vi "Modify Dequeue Cmds to Requested Node Size.vi"(7 "VI to Code Relative Path":string="IONode\\DLULayer\\Dequeue Cmds From Nodes.vi", 8 "Error In":errorcluster, 10 "NumCasesToAdd":i32=1, 11 "Source Root Path":path=path "C:/Users/kvemishe/Downloads/IONode/DLULayer/Dequeue Cmds From Nodes.vi") -> (0 "Error Out":errorcluster, 1 "Found Object?":bool, 3 "Source Root Path Out":path=path "C:/Users/kvemishe/Downloads/IONode/DLULayer/Dequeue Cmds From Nodes.vi")   [LabVIEW 2014]
doc: "This VI scripts the deque commands VI for the IO Node Engine"
uses:
  <vilib>/Utility/traverseref.llb/TRef TravTarget.ctl
  <vilib>/Utility/traverseref.llb/VI Scripting - Traverse.lvlib
panel:
  out "NumCasesFound":i32
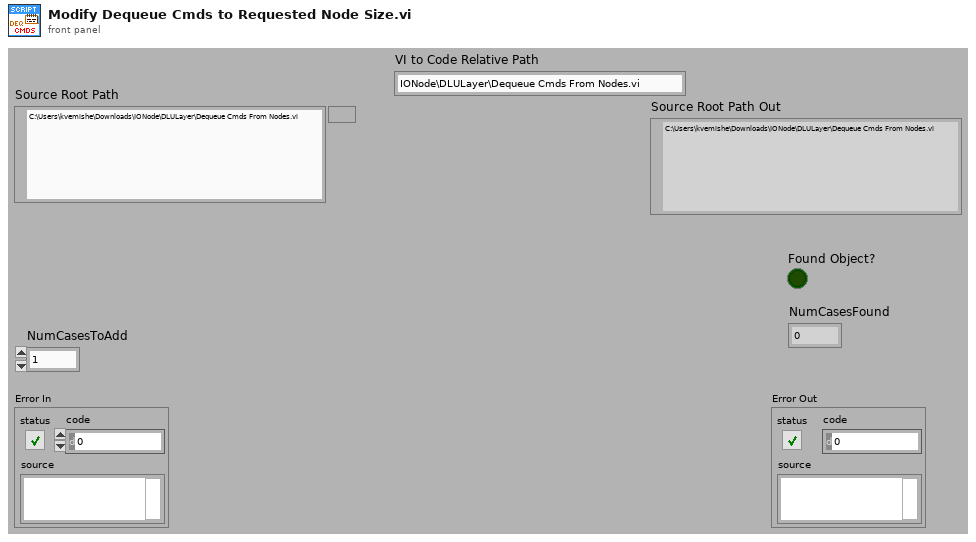
[diagram p1: front panel]
types:
  T1 = typedef "TRef TravTarget.ctl" = enum16{"FP", "BD", "Other"}
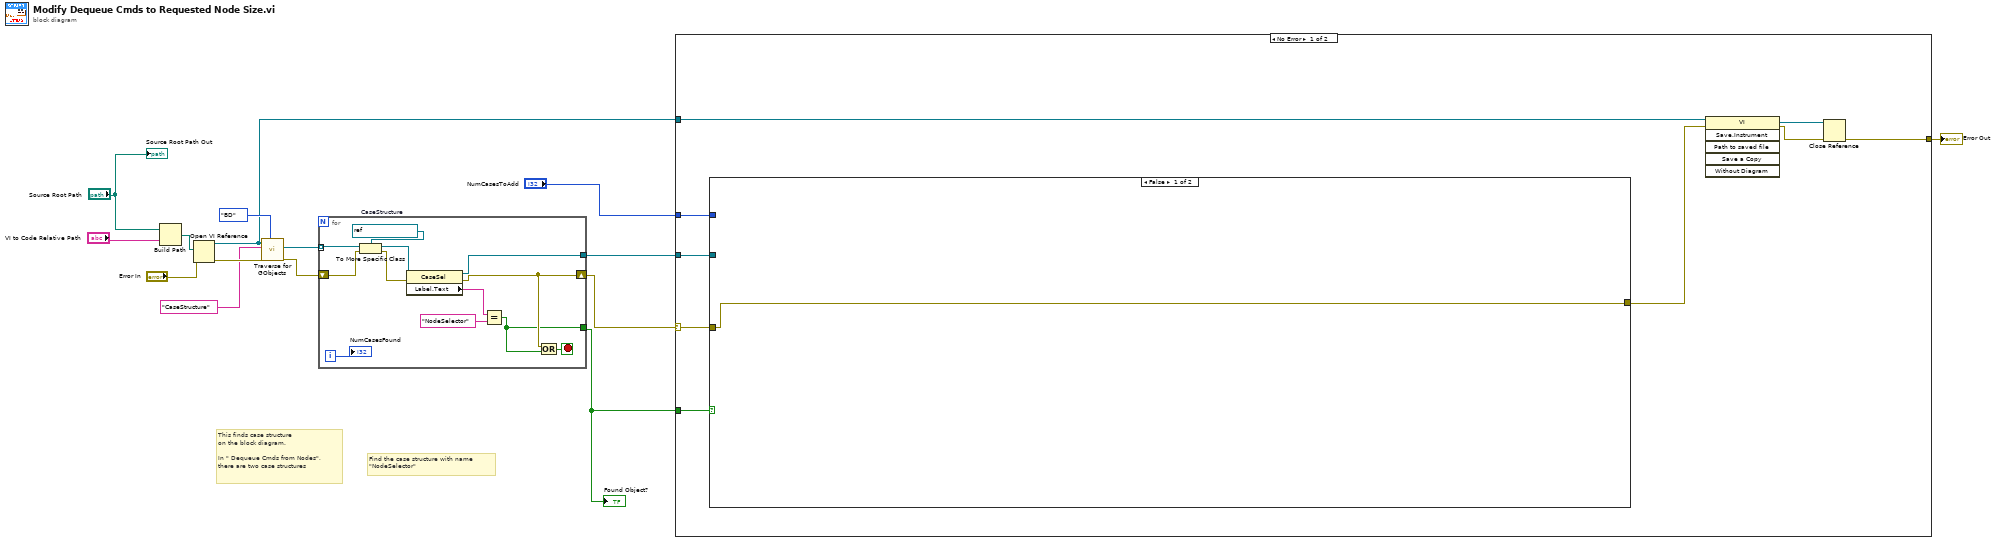
[diagram p0: block diagram]
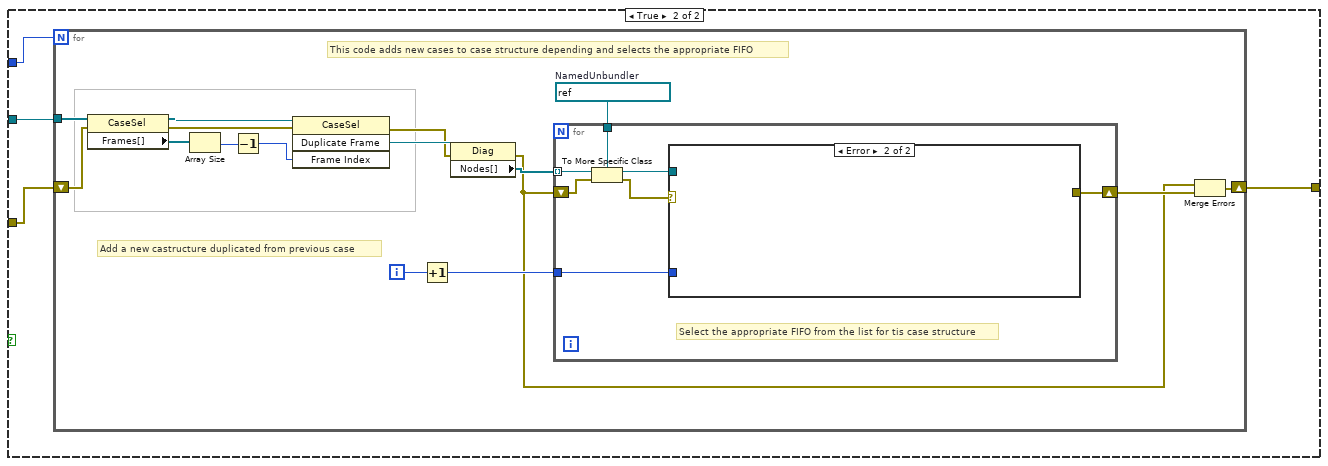
[diagram p2: hidden frame]
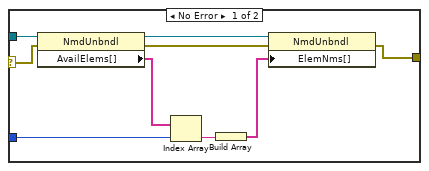
[diagram p3: hidden frame]
diagram:
  # "Find the case structure with name\n\"NodeSelector\""
  # "This finds case structure\non the block diagram.\n\nIn \" Dequeue Cmds from Nodes\",\nthere are two case structures"
  n1 = Build Path(base path="Source Root Path", name or relative path="VI to Code Relative Path") -> (appended path=w3:path)
  n2 = Open VI Reference(vi path=w3, error in (no error)="Error In") -> (vi reference=w6:refnum<vi>, error out=w14:errorcluster)  [unwired: 4 in]
  n3 = call <vilib>:"Traverse for GObjects.vi"("Traverse Target"=TRef_TravTarget."BD", "error in (no error)"=w14, "Class Name"="CaseStructure", "VI Refnum"=w6) -> ("error out"=w11:errorcluster, "References"=w12:refnum<vi>[])  [unwired: 4 in, 2 out]
  n4 = for {
    tunnel: w12 -> [w27] mode=indexing
    shift-right: [w19] -> w9
    shift-left: w11 -> [w25]
    tunnel: [w18] -> w8
    tunnel: [w17] -> w10
    i -> [w16]
    stop <- w20 stop-if-true
    w26 = refnum<vi> refnum  # CaseStructure
    n5 = To More Specific Class(target class=w26, reference=w27, error in=w25) -> (specific class reference=w24:refnum<vi>, error out=w23:errorcluster)
    n6 = property class="CaseSel"(reference=w24, error in=w23) -> (reference out=w17:refnum<vi>, error out=w19:errorcluster, "Label.Text"=w22:string)
    n7 = Equal?(x=w22, y="NodeSelector") -> (x = y?=w18:bool)
    n8 = Or(x=w19, y=w18) -> (x .or. y?=w20:bool)
    "NumCasesFound" <- w16
  }
  "Found Object?" <- w8
  n9 = case shown="No Error" w9 {
    selector: w9 -> [w33 w74]
    tunnel: w10 -> [w36 _]
    tunnel: w8 -> [w35 _]
    tunnel: "NumCasesToAdd" -> [w34 _]
    tunnel: w6 -> [w29 _]
    tunnel: [w28 w74] -> w4
    frame No Error {
      n10 = case shown="False" w35 {
        tunnel: w36 -> [_ w41]
        tunnel: w34 -> [_ w40]
        tunnel: w33 -> [w37 w39]
        tunnel: [w37 w38] -> w30
        frame False {
        }
        frame True {
          n11 = for {
            N: w40 -> [_]
            tunnel: w41 -> [w48]
            shift-right: [w44] -> w38
            shift-left: w39 -> [w45]
            i -> [w47]
            w50 = refnum<vi> refnum  # NamedUnbundler
            # "Add a new castructure duplicated from previous case"
            # "This code adds new cases to case structure depending and selects the appropriate FIFO"
            n12 = property class="CaseSel"(reference=w48, error in=w45) -> (reference out=w57:refnum<vi>, error out=w56:errorcluster, "Frames[]"=w55:refnum<vi>[])
            n13 = Array Size(array=w55) -> (size(s)=w54:i32)
            n14 = Decrement(x=w54) -> (x-1=w53:i32)
            n15 = invoke class="CaseSel" method="Duplicate Frame"(reference=w57, error in=w56, "Frame Index"=w53) -> (error out=w46:errorcluster, "Duplicate Frame"=w52:refnum<vi>)  [unwired: 1 in, 2 out]
            n16 = Increment(x=w47) -> (x+1=w49:i32)
            n17 = property class="Diag"(reference=w52, error in=w46) -> (error out=w42:errorcluster, "Nodes[]"=w51:refnum<vi>[])  [unwired: 1 out]
            n18 = for {
              tunnel: w51 -> [w64] mode=indexing
              tunnel: w50 -> [w63]
              tunnel: w49 -> [w60]
              shift-right: [w59] -> w43
              shift-left: w42 -> [w58]
              # "Select the appropriate FIFO from the list for tis case structure"
              n19 = To More Specific Class(target class=w63, reference=w64, error in=w58) -> (specific class reference=w61:refnum<vi>, error out=w62:errorcluster)
              n20 = case shown="Error" w62 {
                selector: w62 -> [w72 _]
                tunnel: w61 -> [w73 _]
                tunnel: w60 -> [w67 _]
                tunnel: [w65 _] -> w59
                frame No Error {
                  n21 = property class="NmdUnbndl"(reference=w73, error in=w72) -> (reference out=w71:refnum<vi>, error out=w66:errorcluster, "AvailElems[]"=w70:string[])
                  n22 = Index Array(array=w70, index=w67) -> (element=w69:string)
                  n23 = Build Array(w69) -> (w68:string[])
                  n24 = property class="NmdUnbndl"(reference=w71, error in=w66, "ElemNms[]"=w68) -> (error out=w65:errorcluster)  [unwired: 1 out]
                }
                frame Error {
                }
              }
            }
            n25 = Merge Errors(w42, w43) -> (w44:errorcluster)
          }
        }
      }
      n26 = invoke class="VI" method="Save.Instrument"(reference=w29, error in=w30) -> (reference out=w32:refnum<vi>, error out=w31:errorcluster)  [unwired: 4 in, 4 out]
      n27 = Close Reference(reference=w32, error in (no error)=w31) -> (error out=w28:errorcluster)
    }
    frame Error {
    }
  }
  "Error Out" <- w4
  "Source Root Path Out" <- "Source Root Path"
